vi "LoadData (SubVI).vi"(8 "error in (no error)":errorcluster, 10 "VISA resource name out":refnum<visa-resource-name>, 11 "Full Text File":u8[](array[numeric])) -> (0 "error out":errorcluster, 1 "CheckSum Data":u16 format="%.0x", 2 "CheckSum DataB":u16 format="%.0x", 3 "Num of Data packet":i32, 5 "Timeout?":bool)   [LabVIEW 2017]
panel:
  out "Array 4":u16[][](array[numeric]) format="%.0x"
  out "Array 3":u16[][](array[numeric]) format="%.0x"
  out "Array 2":bool[](array[boolean])
  out "Array":bool[][](array[boolean])
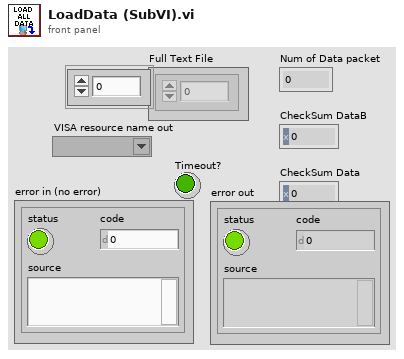
[diagram p1: front panel]
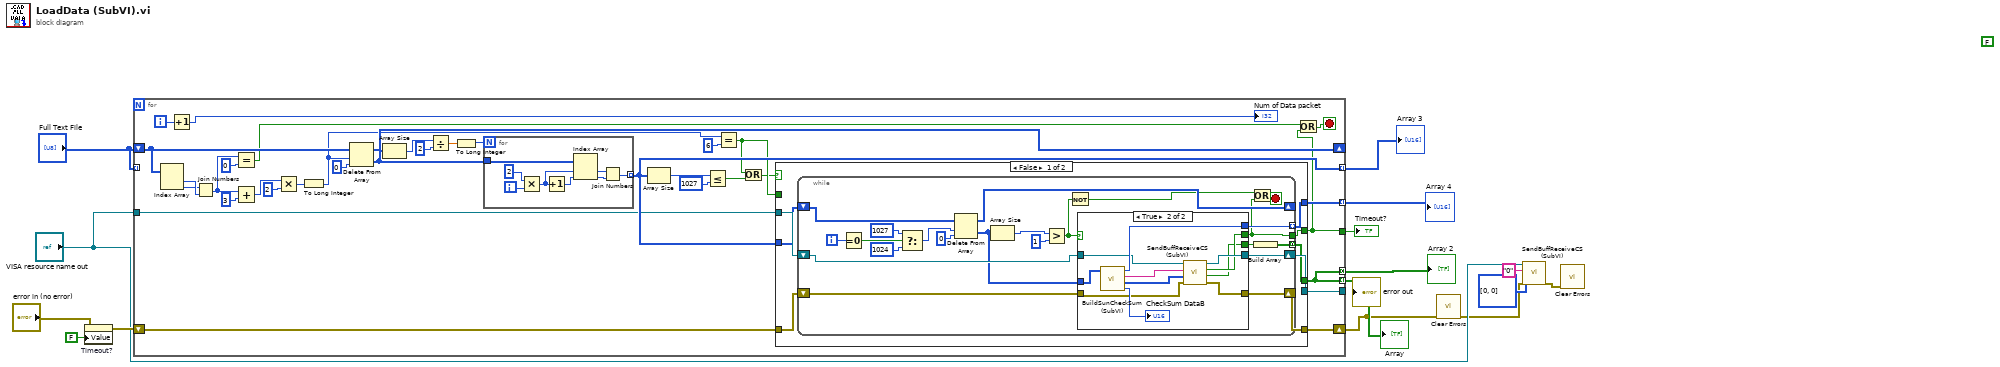
[diagram p0: block diagram]
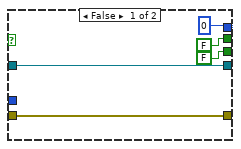
[diagram p2: hidden frame]
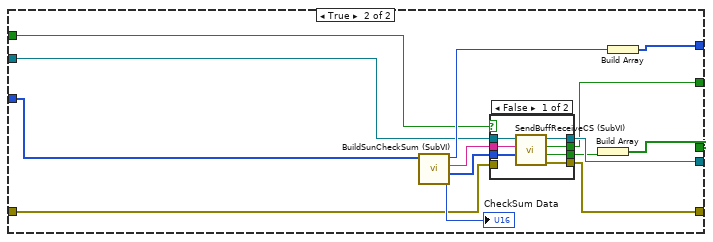
[diagram p3: hidden frame]
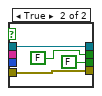
[diagram p4: hidden frame]
diagram:
  (unwired) FALSE
  n1 = property on="Timeout?" class="Bool (strict)"(error in="error in (no error)", "Value"=FALSE ("Timeout?")) -> (error out=w9:errorcluster)  [unwired: 1 in, 1 out]
  n2 = for {
    shift-right: [w40] -> _
    shift-left: "Full Text File" -> [w50]
    tunnel: [w33] -> w11 mode=indexing
    tunnel: "VISA resource name out" -> [w32]
    tunnel: [w29] -> _
    tunnel: [w20] -> w12 mode=concatenating
    tunnel: [w27] -> w10 mode=indexing
    shift-right: [w28] -> w3
    shift-left: w9 -> [w21]
    tunnel: [w20] -> w13 mode=indexing
    tunnel: "Full Text File" -> [_] mode=indexing
    tunnel: [w16] -> w14
    i -> [w41]
    stop <- w17 stop-if-true
    n3 = Index Array(array=w50) -> (element #1=w49:u8, element #2=w48:u8)  [unwired: 2 in]
    n4 = Increment(x=w41) -> (x+1=→"Num of Data packet":i32)
    n5 = Join Numbers(hi=w48, lo=w49) -> ((hi.lo)=w23:u16)
    n6 = Equal?(x=w23, y=u16 0) -> (x = y?=w19:bool)
    n7 = Add(x=w23, y=u32 3) -> (x+y=w46:u32)
    n8 = Multiply(x=w46, y=u32 2) -> (x*y=w44:u32)
    n9 = To Long Integer(number=w44) -> (32bit integer=w24:i32)
    n10 = Delete From Array(array=w50, length=w24, index=0) -> (deleted portion=w25:u8[], array with subset deleted=w40:u8[])
    n11 = Array Size(array=w25) -> (size(s)=w37:i32)
    n12 = Divide(x=w37, y=2) -> (x/y=w39:dbl)
    n13 = To Long Integer(number=w39) -> (32bit integer=w36:i32)
    n14 = for {
      N: w36 -> [_]
      tunnel: w25 -> [w126]
      tunnel: [w122] -> w33 mode=indexing
      i -> [w125]
      n15 = Multiply(x=2, y=w125) -> (x*y=w128:i32)
      n16 = Increment(x=w128) -> (x+1=w129:i32)
      n17 = Index Array(array=w126, index #1=w128, index #2=w129) -> (element #1=w124:u8, element #2=w123:u8)
      n18 = Join Numbers(hi=w124, lo=w123) -> ((hi.lo)=w122:u16)
    }
    n19 = Array Size(array=w33) -> (size(s)=w35:i32)
    n20 = Less Or Equal?(x=w35, y=1027) -> (x <= y?=w30:bool)
    n21 = Equal?(x=w24, y=6) -> (x = y?=w22:bool)
    n22 = Or(x=w22, y=w30) -> (x .or. y?=w18:bool)
    n23 = case shown="False" w18 {
      tunnel: w21 -> [w55 w97]
      tunnel: w32 -> [w58 w105]
      tunnel: [w57 w101] -> w28
      tunnel: [w56 w102] -> w29
      tunnel: w33 -> [w53 w110]
      tunnel: [w54 w109] -> w20
      tunnel: [w52 w107] -> w27
      tunnel: w22 -> [_ w98]
      tunnel: [w51 w99] -> w16
      frame False {
        n24 = while {
          tunnel: [w62] -> w54 mode=concatenating
          shift-right: [w79] -> w56
          shift-left: w58 -> [w80]
          shift-right: [w63] -> w57
          shift-left: w55 -> [w78]
          shift-right: [w71] -> _
          shift-left: w53 -> [w77]
          tunnel: [w70] -> w52 mode=indexing
          tunnel: [w59] -> w51
          i -> [w69]
          stop <- w60 stop-if-true
          n25 = Equal To 0?(x=w69) -> (x = 0?=w68:bool)
          n26 = Select(t=1027 ("length"), s=w68, f=1024 ("length")) -> (s? t:f=w65:i32)
          n27 = Delete From Array(array=w77, length=w65, index=0) -> (deleted portion=w72:u16[], array with subset deleted=w71:u16[])
          n28 = Array Size(array=w72) -> (size(s)=w75:i32)
          n29 = Greater?(x=w75, y=1) -> (0:w73:bool)
          n30 = Not(x=w73) -> (.not. x?=w61:bool)
          n31 = case shown="True" w73 {
            tunnel: w80 -> [w83 w93]
            tunnel: [w85 w86] -> w63
            tunnel: [w83 w89] -> w79
            tunnel: w78 -> [w85 w90]
            tunnel: [FALSE w87] -> w64
            tunnel: w72 -> [_ w94]
            tunnel: [u16 0 ("Numeric") w95] -> w70
            tunnel: [FALSE w88] -> w59
            frame False {
            }
            frame True {
              n32 = call "BuildSunCheckSum (SubVI).vi"("Array in"=w94) -> ("CheckSum DataB"=→"CheckSum DataB":u16, "Buff Out"=w91:u8[], 2:"ExpectedCheckSum"=w92:string, 3:"ExpectedCheckSum"=w95:u16)  [unwired: 6 in]
              n33 = call "SendBuffReceiveCS (SubVI).vi"("error in (no error)"=w90, "Array in"=w91, "ExpectedCheckSum"=w92, "VISA Refnum in"=w93) -> ("error out"=w86:errorcluster, "CorrectCheckSum?"=w87:bool, "Timeout?"=w88:bool, "VISA Refnum out"=w89:refnum<visa-resource-name>)  [unwired: 4 in]
            }
          }
          n34 = Or(x=w61, y=w59) -> (x .or. y?=w60:bool)
          n35 = Build Array(w64) -> (w62:bool[])
        }
      }
      frame True {
        n36 = call "BuildSunCheckSum (SubVI).vi"("Array in"=w110) -> ("CheckSum DataB"=→"CheckSum Data":u16, "Buff Out"=w104:u8[], 2:"ExpectedCheckSum"=w103:string, 3:"ExpectedCheckSum"=w108:u16)  [unwired: 6 in]
        n37 = case shown="False" w98 {
          tunnel: w105 -> [w117 w121]
          tunnel: w104 -> [w116 _]
          tunnel: w103 -> [w111 _]
          tunnel: [w115 w121] -> w102
          tunnel: [w114 w120] -> w101
          tunnel: [w113 FALSE ("CorrectCheckSum?")] -> w100
          tunnel: [w112 FALSE ("CorrectCheckSum?")] -> w99
          tunnel: w97 -> [_ w120]
          frame False {
            n38 = call "SendBuffReceiveCS (SubVI).vi"("Array in"=w116, "ExpectedCheckSum"=w111, "VISA Refnum in"=w117) -> ("error out"=w114:errorcluster, "CorrectCheckSum?"=w113:bool, "Timeout?"=w112:bool, "VISA Refnum out"=w115:refnum<visa-resource-name>)  [unwired: 5 in]
          }
          frame True {
          }
        }
        n39 = Build Array(w100) -> (w109:bool[])
        n40 = Build Array(w108) -> (w107:u16[])
      }
    }
    n41 = Or(x=w19, y=w16) -> (x .or. y?=w17:bool)
  }
  "Timeout?" <- w14
  "Array" <- w13
  "Array 2" <- w12
  "Array 3" <- w11
  "Array 4" <- w10
  "error out" <- w3
  n42 = call <vilib>:"Clear Errors.vi"("error in (no error)"=w3) -> ("error out"=w2:errorcluster)  [unwired: 5 in, 1 out]
  n43 = call "SendBuffReceiveCS (SubVI).vi"("error in (no error)"=w2, "Array in"=u8[] [0, 0], "ExpectedCheckSum"="0", "VISA Refnum in"="VISA resource name out") -> ("error out"=w1:errorcluster)  [unwired: 4 in, 3 out]
  n44 = call <vilib>:"Clear Errors.vi"("error in (no error)"=w1) -> ()  [unwired: 5 in, 2 out]
